vi "meas_cycle_TD_FFT.vi"(2 "PSG freq offset":dbl=0.0003 caption="freq. offset (Hz)" min=0.00025 max=67.0 step=1e-06 format="%#.12p", 3 "time domain array":dbl[](array[numeric]), 4 "dt":dbl, 5 "current frequency":dbl) -> (0 "output time domain signal":waveform(dbl), 1 "output spectrum":T1)   [LabVIEW 2012]
doc: "converts the time domain data to freq. domain data and corrects the frequency offset. \n\nFurthermore, the DC component is deleted from the freq. domain signal."
uses:
  <vilib>/measure/NI_MAPro.lvlib
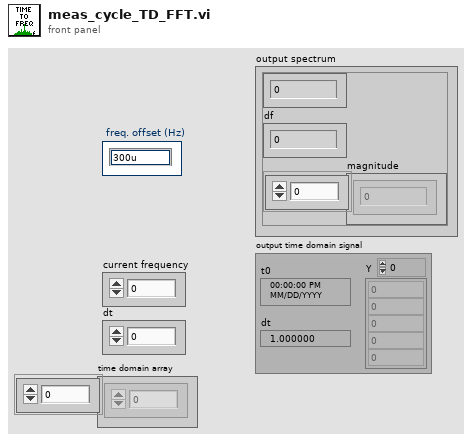
[diagram p1: front panel]
types:
  T1 = cluster{"Numeric Control":dbl, "df":dbl, "magnitude":dbl[]}
  T2 = cluster{dbl, "df":dbl, "power spectrum (V^2 rms)":dbl[]}
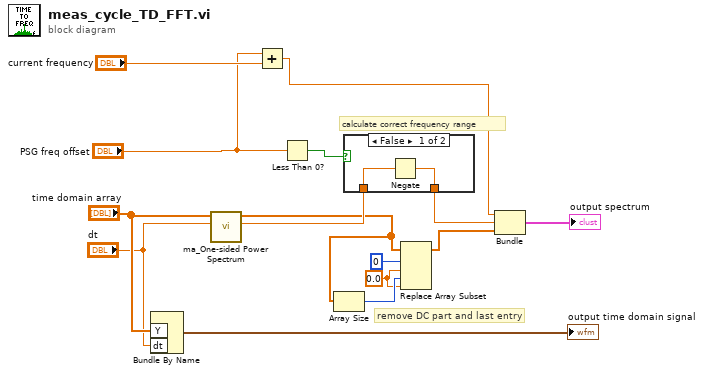
[diagram p0: block diagram]
diagram:
  w13 = 0.0 ("new element/subarray")
  # "calculate correct frequency range"
  # "remove DC part and last entry"
  n1 = Bundle By Name("Y"="time domain array", "dt"="dt") -> (→"output time domain signal":waveform(dbl))  [unwired: 1 in]
  n2 = call <vilib>:"ma_One-sided Power Spectrum.vi"("dt"="dt", "signal (V)"="time domain array") -> ("df"=w2:dbl, "power spectrum (V^2 rms)"=w1:dbl[])  [unwired: 1 in, 7 out]
  n3 = Add(x="PSG freq offset", y="current frequency") -> (x+y=w6:dbl)
  n4 = Less Than 0?(x="PSG freq offset") -> (x < 0?=w9:bool)
  n5 = Array Size(array=w1) -> (size(s)=w14:i32)
  n6 = case shown="False" w9 {
    tunnel: w2 -> [w17 w18]
    tunnel: [w16 w18] -> w10
    frame False {
      n7 = Negate(x=w17) -> (-x=w16:dbl)
    }
    frame True {
    }
  }
  n8 = Replace Array Subset(array=w1, new element #1=w13, index #1=0 ("index"), new element #2=w13, index #2=w14) -> (w12:dbl[])
  n9 = Bundle(w6, "df"=w10, "power spectrum (V^2 rms)"=w12) -> (→"output spectrum":T2)  [unwired: 1 in]
